vi "monitorización de variables.vi"() -> ()   [LabVIEW 2019]
uses:
  <vilib>/NI/Modbus Library/API/Wrapper/Create Serial Master.vi
  <vilib>/NI/Modbus Library/API/Master/Modbus Master.lvclass
  <vilib>/NI/Modbus Library/API/Wrapper/API Main.lvlib
panel:
  in  "Cargas Manuales":bool
  out "Repetición":dbl
  out "Frecuencia Real VFD":dbl
  in  "Mediciones automaticas":bool
  out "Frecuencia VFD":dbl
  out "Tiempo Transcurrido entre frecuencias del VFD":dbl
  out "Torque Generador":dbl
  out "Velocidad medida (rpm)":dbl
  out "Frecuencia de rotación":dbl
  out "Voltaje VFD":dbl
  out "Corriente VFD":dbl
  out "Corriente VFD":dbl(knob) scale=0.0..2.0
  out "Voltaje VFD":dbl(knob) scale=0.0..220.0
  in  "Cargas Automáticas":bool=TRUE
  out "tiempo de control cargas":dbl
  out "Carga Electrica Automática":dbl
  in  "Apagar Ejecución":bool=TRUE
  in  "Control de Caragas":T1(ring)
  in  "VFD":bool
  in  "Frequency":dbl(knob) step=1.0 scale=0.0..75.0
  in  "stop":bool
  in  "Baud rate":u32=9600
  in  "Puerto":refnum<visa-resource-name>
  in  "Motor a analizar":dbl
  out "Torque":dbl
  out "Torque":dbl(knob) scale=-10.0..10.0
  out "Corriente generado":dynamicdata(graph)
  out "Corriente":dbl
  out "Voltaje":dbl
  out "Corriente RMS":dbl(knob) scale=0.0..2.0
  out "Voltaje generado":dynamicdata(graph)
  out "Voltaje RMS":dbl(knob) scale=0.0..230.0
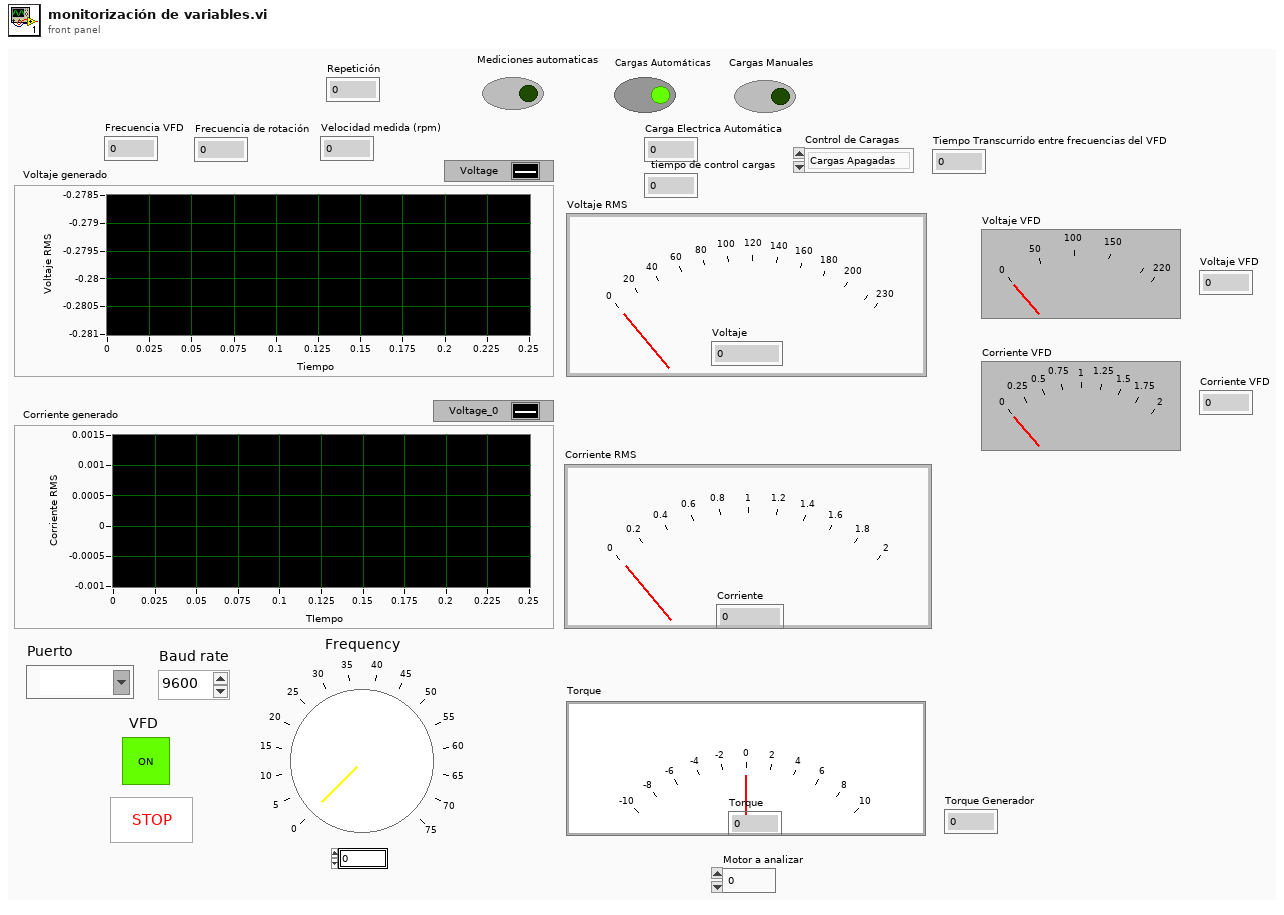
[diagram p1: front panel]
types:
  T1 = enum16{"Cargas Apagadas", "Activar Primer Carga", "Activar Segunda Carga", "Activar Ambas Cargas"}
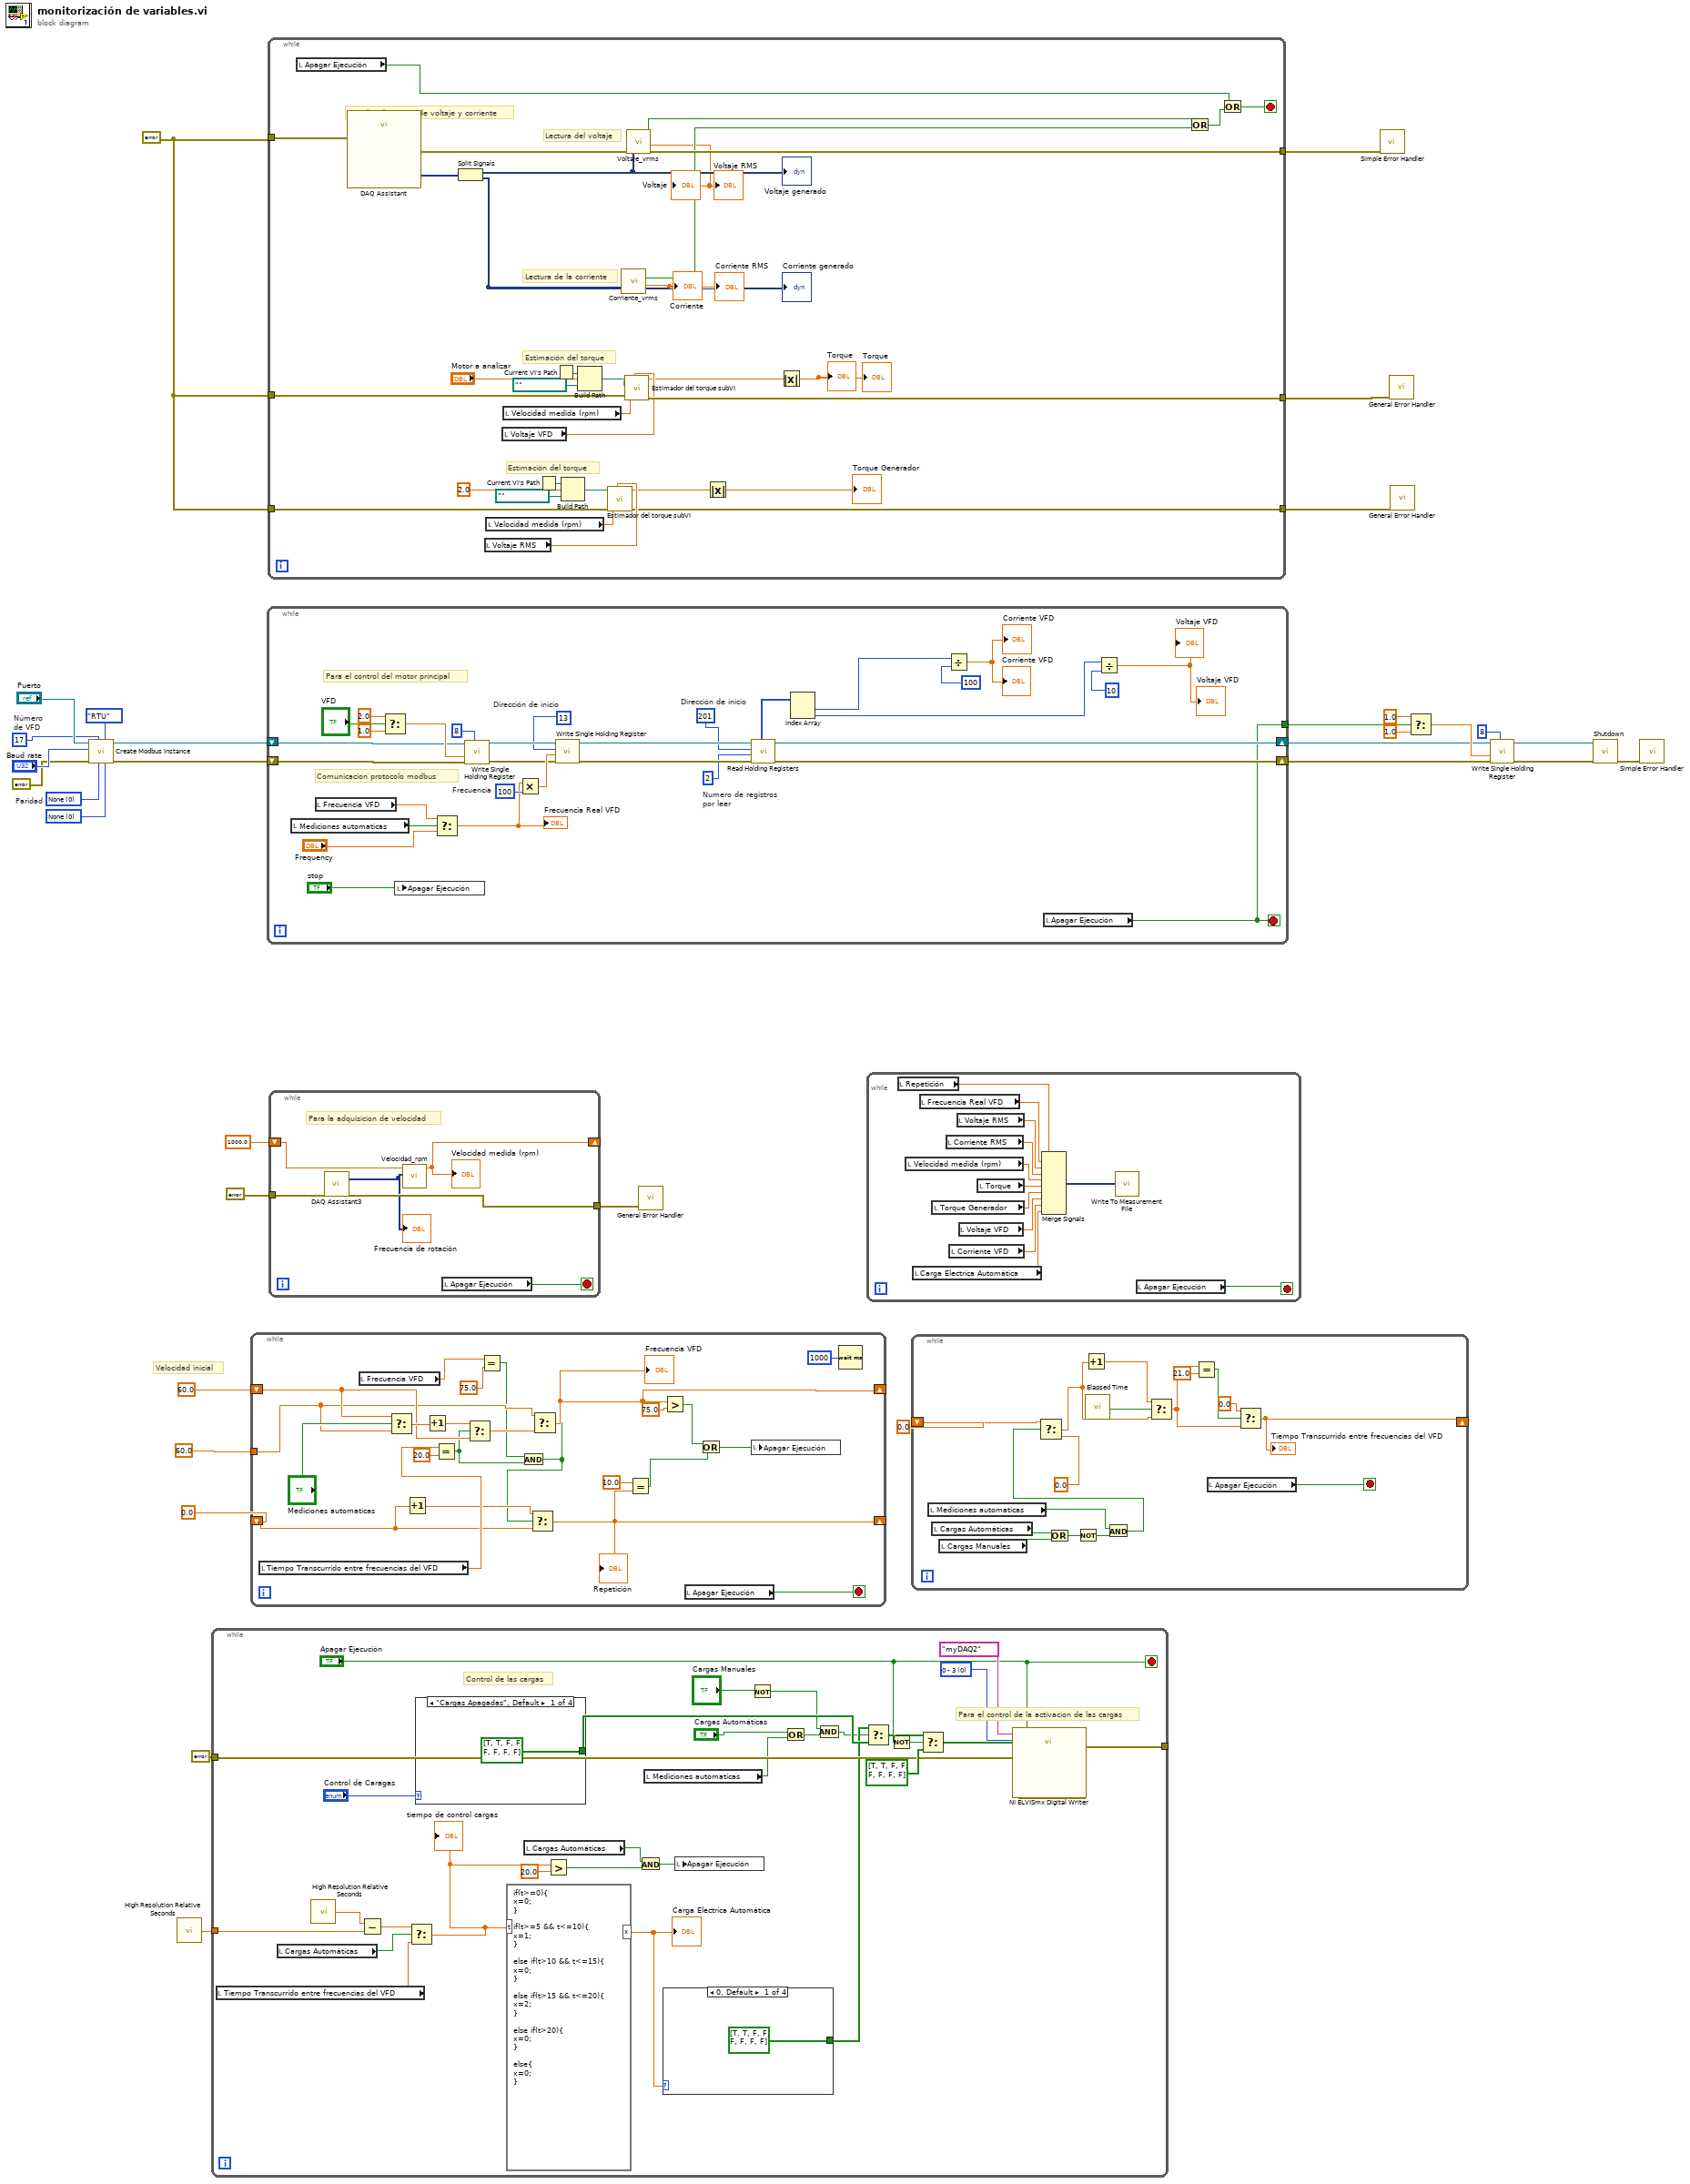
[diagram p0: block diagram]
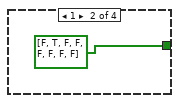
[diagram p2: hidden frame]
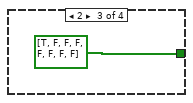
[diagram p3: hidden frame]
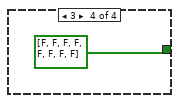
[diagram p4: hidden frame]
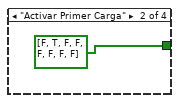
[diagram p5: hidden frame]
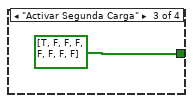
[diagram p6: hidden frame]
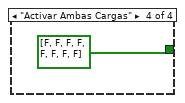
[diagram p7: hidden frame]
diagram:
  w26 = u16 0 items=["None", "Odd", "Even", "Mark", "Space"]  # Paridad
  w27 = u16 0 items=["None", "XON/XOFF", "RTS/CTS", "XON/XOFF & RTS/CTS", "DTR/DSR", "XON/XOFF & DTR/DSR"] ("flow control (none)")
  w25 = u8 17  # Número de VFD
  w11 = errorcluster {"status"=FALSE, "code"=0, "source"=""} ("error in")
  # "Velocidad inicial"
  n1 = call-poly <vilib>:"Create Modbus Instance.vi"("flow control (none)"=w27, "serial type"=enum16{"RTU", "ASCII"}."RTU", "parity (even)"=w26, "unit ID"=w25, "error in"=errorcluster {"status"=FALSE, "code"=0, "source"=""}, "baud rate"="Baud rate", "VISA resource name"="Puerto") -> ("error out"=w9:errorcluster, "serial master instance"=w10:refnum<class "Modbus Master.lvclass">)  [unwired: 3 in]
  n2 = call <vilib>:"High Resolution Relative Seconds.vi"() -> ("relative seconds"=w15:dbl)
  n3 = while {
    tunnel: errorcluster {"status"=FALSE, "code"=0, "source"=""} ("error in") -> [w55]
    tunnel: [w54] -> _
    tunnel: w15 -> [w52]
    stop <- "Apagar Ejecución" stop-if-true
    w56 = u16 0 items=["0 - 3", "4 - 7", "0 - 7"] ("myDAQ Lines to Write")
    # "Control de las cargas"
    # "Para el control de la activacion de las cargas"
    n4 = local read "Tiempo Transcurrido entre frecuencias del VFD"() -> (w39:dbl)
    n5 = local read "Cargas Automáticas"() -> (w40:bool)
    n6 = call <vilib>:"High Resolution Relative Seconds.vi"() -> ("relative seconds"=w51:dbl)
    n7 = Subtract(x=w51, y=w52) -> (x-y=w42:dbl)
    n8 = Select(t=w42, s=w40, f=w39) -> (s? t:f=w41:dbl)
    "tiempo de control cargas" <- w41
    n9 = case shown="\"Cargas Apagadas\", Default" "Control de Caragas" {
      tunnel: [bool[] [TRUE, TRUE, FALSE, FALSE, FALSE, FALSE, FALSE, FALSE] ("DO Lines") bool[] [FALSE, TRUE, FALSE, FALSE, FALSE, FALSE, FALSE, FALSE] ("DO Lines") bool[] [TRUE, FALSE, FALSE, FALSE, FALSE, FALSE, FALSE, FALSE] ("DO Lines") bool[] [FALSE, FALSE, FALSE, FALSE, FALSE, FALSE, FALSE, FALSE] ("DO Lines")] -> w49
      frame "Cargas Apagadas", Default {
      }
      frame "Activar Primer Carga" {
      }
      frame "Activar Segunda Carga" {
      }
      frame "Activar Ambas Cargas" {
      }
    }
    n10 = formula code="if(t>=0){\nx=0;\n}\n\nif(t>=5 && t<=10){\nx=1;\n}\n\nelse if(t>10 && t<=15){\nx=0;\n}\n\nelse if(t>15 && t<=20){\nx=2;\n}\n\nelse if(t>20){\nx=0;\n}\n\nelse{\nx=0;\n}"("t"=w41) -> ("x"=w50:dbl)
    "Carga Electrica Automática" <- w50
    n11 = local read "Cargas Automáticas"() -> (w43:bool)
    n12 = Greater?(x=w41, y=20.0) -> (0:w44:bool)
    n13 = And(x=w43, y=w44) -> (x .and. y?=w45:bool)
    n14 = local read "Mediciones automaticas"() -> (w38:bool)
    n15 = case shown="0, Default" w50 {
      tunnel: [bool[] [TRUE, TRUE, FALSE, FALSE, FALSE, FALSE, FALSE, FALSE] ("DO Lines") bool[] [FALSE, TRUE, FALSE, FALSE, FALSE, FALSE, FALSE, FALSE] ("DO Lines") bool[] [TRUE, FALSE, FALSE, FALSE, FALSE, FALSE, FALSE, FALSE] ("DO Lines") bool[] [FALSE, FALSE, FALSE, FALSE, FALSE, FALSE, FALSE, FALSE] ("DO Lines")] -> w47
      frame 0, Default {
      }
      frame 1 {
      }
      frame 2 {
      }
      frame 3 {
      }
    }
    n16 = local write "Apagar Ejecución"(w45) -> ()
    n17 = Not(x="Cargas Manuales") -> (.not. x?=w34:bool)
    n18 = Or(x="Cargas Automáticas", y=w38) -> (x .or. y?=w37:bool)
    n19 = And(x=w34, y=w37) -> (x .and. y?=w36:bool)
    n20 = Select(t=w47, s=w36, f=w49) -> (s? t:f=w48:bool[])
    n21 = Not(x="Apagar Ejecución") -> (.not. x?=w60:bool)
    n22 = Select(t=w48, s=w60, f=bool[] [TRUE, TRUE, FALSE, FALSE, FALSE, FALSE, FALSE, FALSE] ("DO Lines")) -> (s? t:f=w57:bool[])
    n23 = call "NI ELVISmx Digital Writer"("Device Name"=tag "myDAQ2", "myDAQ Lines to Write"=w56, "Stop"="Apagar Ejecución", "DO Lines"=w57, "error in"=w55) -> ("error out"=w54:errorcluster)  [unwired: 14 in]
  }
  n24 = while {
    shift-right: [w90] -> _
    shift-left: 60.0 -> [w85]
    tunnel: 60.0 -> [w74]
    shift-right: [w81] -> _
    shift-left: 0.0 -> [w83]
    stop <- w93 stop-if-true
    n25 = local read "Tiempo Transcurrido entre frecuencias del VFD"() -> (w89:dbl)
    n26 = local read "Frecuencia VFD"() -> (w73:dbl)
    n27 = Select(t=w85, s="Mediciones automaticas", f=w74) -> (s? t:f=w92:dbl)
    n28 = Increment(x=w83) -> (x+1=w82:dbl)
    n29 = Increment(x=w92) -> (x+1=w87:dbl)
    n30 = Equal?(x=w89, y=20.0) -> (x = y?=w75:bool)
    n31 = Select(t=w87, s=w75, f=w85) -> (s? t:f=w86:dbl)
    n32 = Equal?(x=w73, y=75.0) -> (x = y?=w71:bool)
    n33 = And(x=w71, y=w75) -> (x .and. y?=w70:bool)
    n34 = Select(t=w82, s=w70, f=w83) -> (s? t:f=w81:dbl)
    "Repetición" <- w81
    n35 = Select(t=w74, s=w70, f=w86) -> (s? t:f=w90:dbl)
    "Frecuencia VFD" <- w90
    n36 = Equal?(x=10.0, y=w81) -> (x = y?=w76:bool)
    n37 = Greater?(x=w90, y=75.0) -> (0:w79:bool)
    n38 = local read "Apagar Ejecución"() -> (w93:bool)
    n39 = Or(x=w79, y=w76) -> (x .or. y?=w78:bool)
    n40 = local write "Apagar Ejecución"(w78) -> ()
    n41 = Wait (ms)(milliseconds to wait=u32 1000) -> ()  [unwired: 1 out]
  }
  n42 = while {
    shift-right: [w101] -> w7
    shift-left: w10 -> [w103]
    shift-right: [w100] -> w8
    shift-left: w9 -> [w102]
    tunnel: [w99] -> w6
    stop <- w99 stop-if-true
    w115 = u16 2  # Numero de registros  por leer
    w114 = u16 201  # Dirección de inicio
    w111 = u16 100  # Frecuencia
    w105 = u16 13  # Dirección de inicio
    # "Comunicacion protocolo modbus"
    # "Para el control del motor principal"
    n43 = local read "Mediciones automaticas"() -> (w98:bool)
    n44 = local read "Frecuencia VFD"() -> (w97:dbl)
    n45 = Select(t=2.0, s="VFD", f=1.0) -> (s? t:f=w113:dbl)
    n46 = local write "Apagar Ejecución"("stop") -> ()
    n47 = Select(t=w97, s=w98, f="Frequency") -> (s? t:f=w95:dbl)
    "Frecuencia Real VFD" <- w95
    n48 = call-dynamic "Write Single Holding Register.vi"("error in"=w102, "register to write"=w113, "address"=u16 8 ("Start"), "Modbus master in"=w103) -> ("error out"=w107:errorcluster, "Modbus master out"=w106:refnum<class "Modbus Master.lvclass">)  [unwired: 6 in]
    n49 = Multiply(x=w95, y=w111) -> (x*y=w112:dbl)
    n50 = call-dynamic "Write Single Holding Register.vi"("error in"=w107, "register to write"=w112, "address"=w105, "Modbus master in"=w106) -> ("error out"=w124:errorcluster, "Modbus master out"=w123:refnum<class "Modbus Master.lvclass">)  [unwired: 6 in]
    n51 = call-dynamic "Read Holding Registers.vi"("error in"=w124, "number of inputs"=w115, "starting address"=w114, "Modbus master in"=w123) -> ("error out"=w100:errorcluster, "register values"=w116:u16[], "Modbus master out"=w101:refnum<class "Modbus Master.lvclass">)  [unwired: 5 in]
    n52 = Index Array(array=w116) -> (element #1=w120:u16, element #2=w117:u16)  [unwired: 2 in]
    n53 = Divide(x=w120, y=u16 100) -> (x/y=→"Corriente VFD" →"Corriente VFD":dbl)
    n54 = local read "Apagar Ejecución"() -> (w99:bool)
    n55 = Divide(x=w117, y=u16 10) -> (x/y=→"Voltaje VFD" →"Voltaje VFD":dbl)
  }
  n56 = while {
    tunnel: w11 -> [w143]
    tunnel: [w157] -> w17
    tunnel: w11 -> [w131]
    tunnel: [w147] -> w32
    tunnel: [w130] -> w5
    tunnel: w11 -> [w129]
    stop <- w142 stop-if-true
    # "Estimación del torque"
    # "Para la adquisición de voltaje y corriente"
    # "Estimación del torque"
    # "Lectura de la corriente"
    # "Lectura del voltaje"
    n57 = local read "Apagar Ejecución"() -> (w138:bool)
    n58 = call "DAQ Assistant"("error in"=w143) -> ("data"=w145:dynamicdata, "error out"=w144:errorcluster)  [unwired: 15 in, 2 out]
    n59 = Split Signals(w145) -> (w156:dynamicdata, w151:dynamicdata)  [unwired: 2 in]
    "Voltaje generado" <- w156
    "Corriente generado" <- w151
    n60 = local read "Voltaje RMS"() -> (w133:dbl)
    n61 = local read "Velocidad medida (rpm)"() -> (w134:dbl)
    n62 = local read "Voltaje VFD"() -> (w140:dbl)
    n63 = local read "Velocidad medida (rpm)"() -> (w141:dbl)
    n64 = Current VI's Path() -> (path=w137:path)
    n65 = Current VI's Path() -> (path=w150:path)
    n66 = Build Path(base path=w137, name or relative path=path "") -> (appended path=w135:path)
    n67 = Build Path(base path=w150, name or relative path=path "") -> (appended path=w148:path)
    n68 = call "Estimador del torque subVI.vi"("Real"=w133, "error in (no error)"=w129, "Real 2"=w134, "Real 3"=2.0 ("Motor a analizar 2"), "appended path"=w135) -> ("error out"=w130:errorcluster, "Numeric"=w126:dbl)  [unwired: 5 in]
    n69 = call "Corriente_vrms.vi"("Dynamic Data"=w151) -> ("Scalar"=→"Corriente RMS" →"Corriente":dbl, "Boolean"=w154:bool)  [unwired: 8 in, 1 out]
    n70 = call "Estimador del torque subVI.vi"("Real"=w140, "error in (no error)"=w131, "Real 2"=w141, "Real 3"="Motor a analizar", "appended path"=w148) -> ("error out"=w147:errorcluster, "Numeric"=w128:dbl)  [unwired: 5 in]
    n71 = call "Voltaje_vrms.vi"("error in (no error)"=w144, "data"=w156) -> ("error out"=w157:errorcluster, "Scalar"=→"Voltaje RMS" →"Voltaje":dbl, "Boolean"=w153:bool)  [unwired: 6 in, 1 out]
    n72 = Absolute Value(x=w126) -> (abs(x)=→"Torque Generador":dbl)
    n73 = Absolute Value(x=w128) -> (abs(x)=→"Torque" →"Torque":dbl)
    n74 = Or(x=w153, y=w154) -> (x .or. y?=w152:bool)
    n75 = Or(x=w138, y=w152) -> (x .or. y?=w142:bool)
  }
  n76 = while {
    shift-right: [w160] -> _
    shift-left: 1000.0 -> [w163]
    tunnel: [w162] -> w12
    tunnel: errorcluster {"status"=FALSE, "code"=0, "source"=""} ("error in") -> [w161]
    stop <- w158 stop-if-true
    # "Para la adquisicion de velocidad"
    n77 = call "DAQ Assistant3"("error in"=w161) -> ("data"=w159:dynamicdata, "error out"=w162:errorcluster)  [unwired: 16 in, 1 out]
    "Frecuencia de rotación" <- w159
    n78 = call "Velocidad_rpm.vi"("data"=w159, "Numeric in"=w163) -> ("Numeric out"=w160:dbl)  [unwired: 9 in]
    "Velocidad medida (rpm)" <- w160
    n79 = local read "Apagar Ejecución"() -> (w158:bool)
  }
  n80 = call <vilib>:"General Error Handler.vi"("error in (no error)"=w12) -> ()  [unwired: 10 in, 5 out]
  n81 = while {
    stop <- w166 stop-if-true
    n82 = local read "Repetición"() -> (w164:dbl)
    n83 = local read "Velocidad medida (rpm)"() -> (w172:dbl)
    n84 = local read "Carga Electrica Automática"() -> (w167:dbl)
    n85 = local read "Frecuencia Real VFD"() -> (w165:dbl)
    n86 = local read "Torque Generador"() -> (w168:dbl)
    n87 = local read "Corriente RMS"() -> (w171:dbl)
    n88 = local read "Corriente VFD"() -> (w175:dbl)
    n89 = local read "Voltaje RMS"() -> (w170:dbl)
    n90 = local read "Voltaje VFD"() -> (w174:dbl)
    n91 = local read "Torque"() -> (w173:dbl)
    n92 = Merge Signals(w164, w165, w170, w171, w172, w173, w168, w174, w175, w167) -> (w169:dynamicdata)
    n93 = call "Write To Measurement File"("Signals"=w169) -> ()  [unwired: 16 in, 3 out]
    n94 = local read "Apagar Ejecución"() -> (w166:bool)
  }
  n95 = while {
    shift-right: [w185] -> _
    shift-left: 0.0 ("t") -> [w183]
    stop <- w186 stop-if-true
    n96 = local read "Mediciones automaticas"() -> (w177:bool)
    n97 = local read "Cargas Automáticas"() -> (w181:bool)
    n98 = local read "Cargas Manuales"() -> (w180:bool)
    n99 = Or(x=w181, y=w180) -> (x .or. y?=w179:bool)
    n100 = Not(x=w179) -> (.not. x?=w178:bool)
    n101 = call "Elapsed Time"() -> ("Time has Elapsed"=w191:bool)  [unwired: 12 in, 7 out]
    n102 = And(x=w177, y=w178) -> (x .and. y?=w176:bool)
    n103 = Select(t=w183, s=w176, f=0.0) -> (s? t:f=w184:dbl)
    n104 = Increment(x=w184) -> (x+1=w192:dbl)
    n105 = Select(t=w192, s=w191, f=w184) -> (s? t:f=w189:dbl)
    n106 = Equal?(x=w189, y=21.0) -> (x = y?=w190:bool)
    n107 = local read "Apagar Ejecución"() -> (w186:bool)
    n108 = Select(t=0.0, s=w190, f=w189) -> (s? t:f=w185:dbl)
    "Tiempo Transcurrido entre frecuencias del VFD" <- w185
  }
  n109 = call <vilib>:"Simple Error Handler.vi"("error in (no error)"=w17) -> ()  [unwired: 4 in, 5 out]
  n110 = call <vilib>:"General Error Handler.vi"("error in (no error)"=w32) -> ()  [unwired: 10 in, 5 out]
  n111 = call <vilib>:"General Error Handler.vi"("error in (no error)"=w5) -> ()  [unwired: 10 in, 5 out]
  n112 = Select(t=1.0, s=w6, f=1.0) -> (s? t:f=w20:dbl)
  n113 = call-dynamic "Write Single Holding Register.vi"("error in"=w8, "register to write"=w20, "address"=u16 8 ("Start"), "Modbus master in"=w7) -> ("error out"=w18:errorcluster, "Modbus master out"=w19:refnum<class "Modbus Master.lvclass">)  [unwired: 6 in]
  n114 = call-dynamic "Shutdown.vi"("error in"=w18, "Modbus master in"=w19) -> ("error out"=w24:errorcluster)  [unwired: 9 in]
  n115 = call <vilib>:"Simple Error Handler.vi"("error in (no error)"=w24) -> ()  [unwired: 4 in, 5 out]
